vi "Change Instrument Identity.vi"(8 "error in (no error)":errorcluster, 9 "Model Number":string, 10 "Manufacturer Identity (1: Keysight)":i32(ring)=1 items=["Agilent", "Keysight"], 11 "VISA resource name":refnum<visa-resource-name>) -> (0 "error out":errorcluster, 3 "VISA resource name out":refnum<visa-resource-name>)   [LabVIEW 2016, in "Agilent N6700 Series.lvlib"]
doc: "Changes the model number and manufacturer identity for compatibility.\n\n<b>Note:</b>\nThis VI only applies to N6700C, N6701C, N6702C and N6705C."
uses:
  <instrlib>/Agilent N6700 Series/Agilent N6700 Series.lvlib
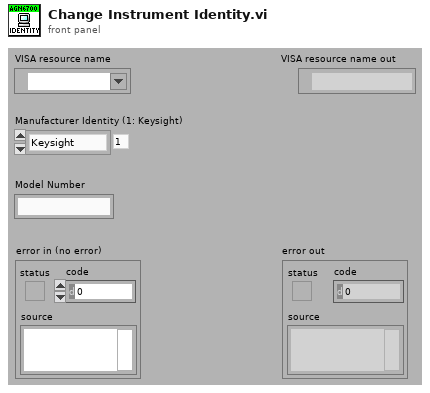
[diagram p1: front panel]
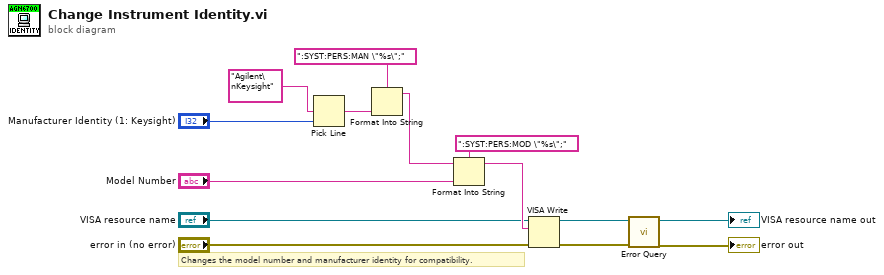
[diagram p0: block diagram]
diagram:
  # "Changes the model number and manufacturer identity for compatibility."
  n1 = Pick Line(multi-line string="Agilent\nKeysight", line index="Manufacturer Identity (1: Keysight)") -> (output string=w2:string)  [unwired: 1 in]
  n2 = Format Into String(format string=":SYST:PERS:MAN \"%s\";", w2) -> (resulting string=w1:string)  [unwired: 2 in, 1 out]
  n3 = Format Into String(format string=":SYST:PERS:MOD \"%s\";", initial string=w1, "Model Number") -> (resulting string=w10:string)  [unwired: 1 in, 1 out]
  n4 = VISA Write(VISA resource name="VISA resource name", write buffer=w10, error in (no error)="error in (no error)") -> (VISA resource name out=w7:refnum<visa-resource-name>, error out=w6:errorcluster)  [unwired: 1 out]
  n5 = call <instrlib>:"Error Query.vi"("VISA resource name"=w7, "error in (no error)"=w6) -> ("VISA resource name out"=→"VISA resource name out":refnum<visa-resource-name>, "error out"=→"error out":errorcluster)  [unwired: 10 in, 2 out]
